vi "PlanetInfo.vi"(8 "error in (no error)":errorcluster) -> (0 "error out":errorcluster, 1 "stop?":bool, 3 "PlanetInfo":T1)   [LabVIEW 2021]
uses:
  <vilib>/Utility/miscctls.llb/LVRectTypeDef.ctl
  <vilib>/Utility/miscctls.llb/LVPoint32TypeDef.ctl
  Typedefs/PlanetInfo.ctl
  <vilib>/Utility/miscctls.llb/LVBoundsTypeDef.ctl
panel:
  out "Coords":T2
  out "Window Bounds":T3
  out "Is Window Dragged?":bool
  in  "Tab":enum32{"Page 1"}(tab)
  in  "Ring gear of teeth":dbl=72.0
  in  "Satelite gear of teeth":dbl=24.0
  in  "Sun gear of teeth":dbl=24.0
  in  "Number of satelites":dbl=3.0
  in  "Save":bool
  out "WindowHandler":bool=TRUE
  out "Komunikat":string caption="Wpisz kod"
  in  "Stop":bool
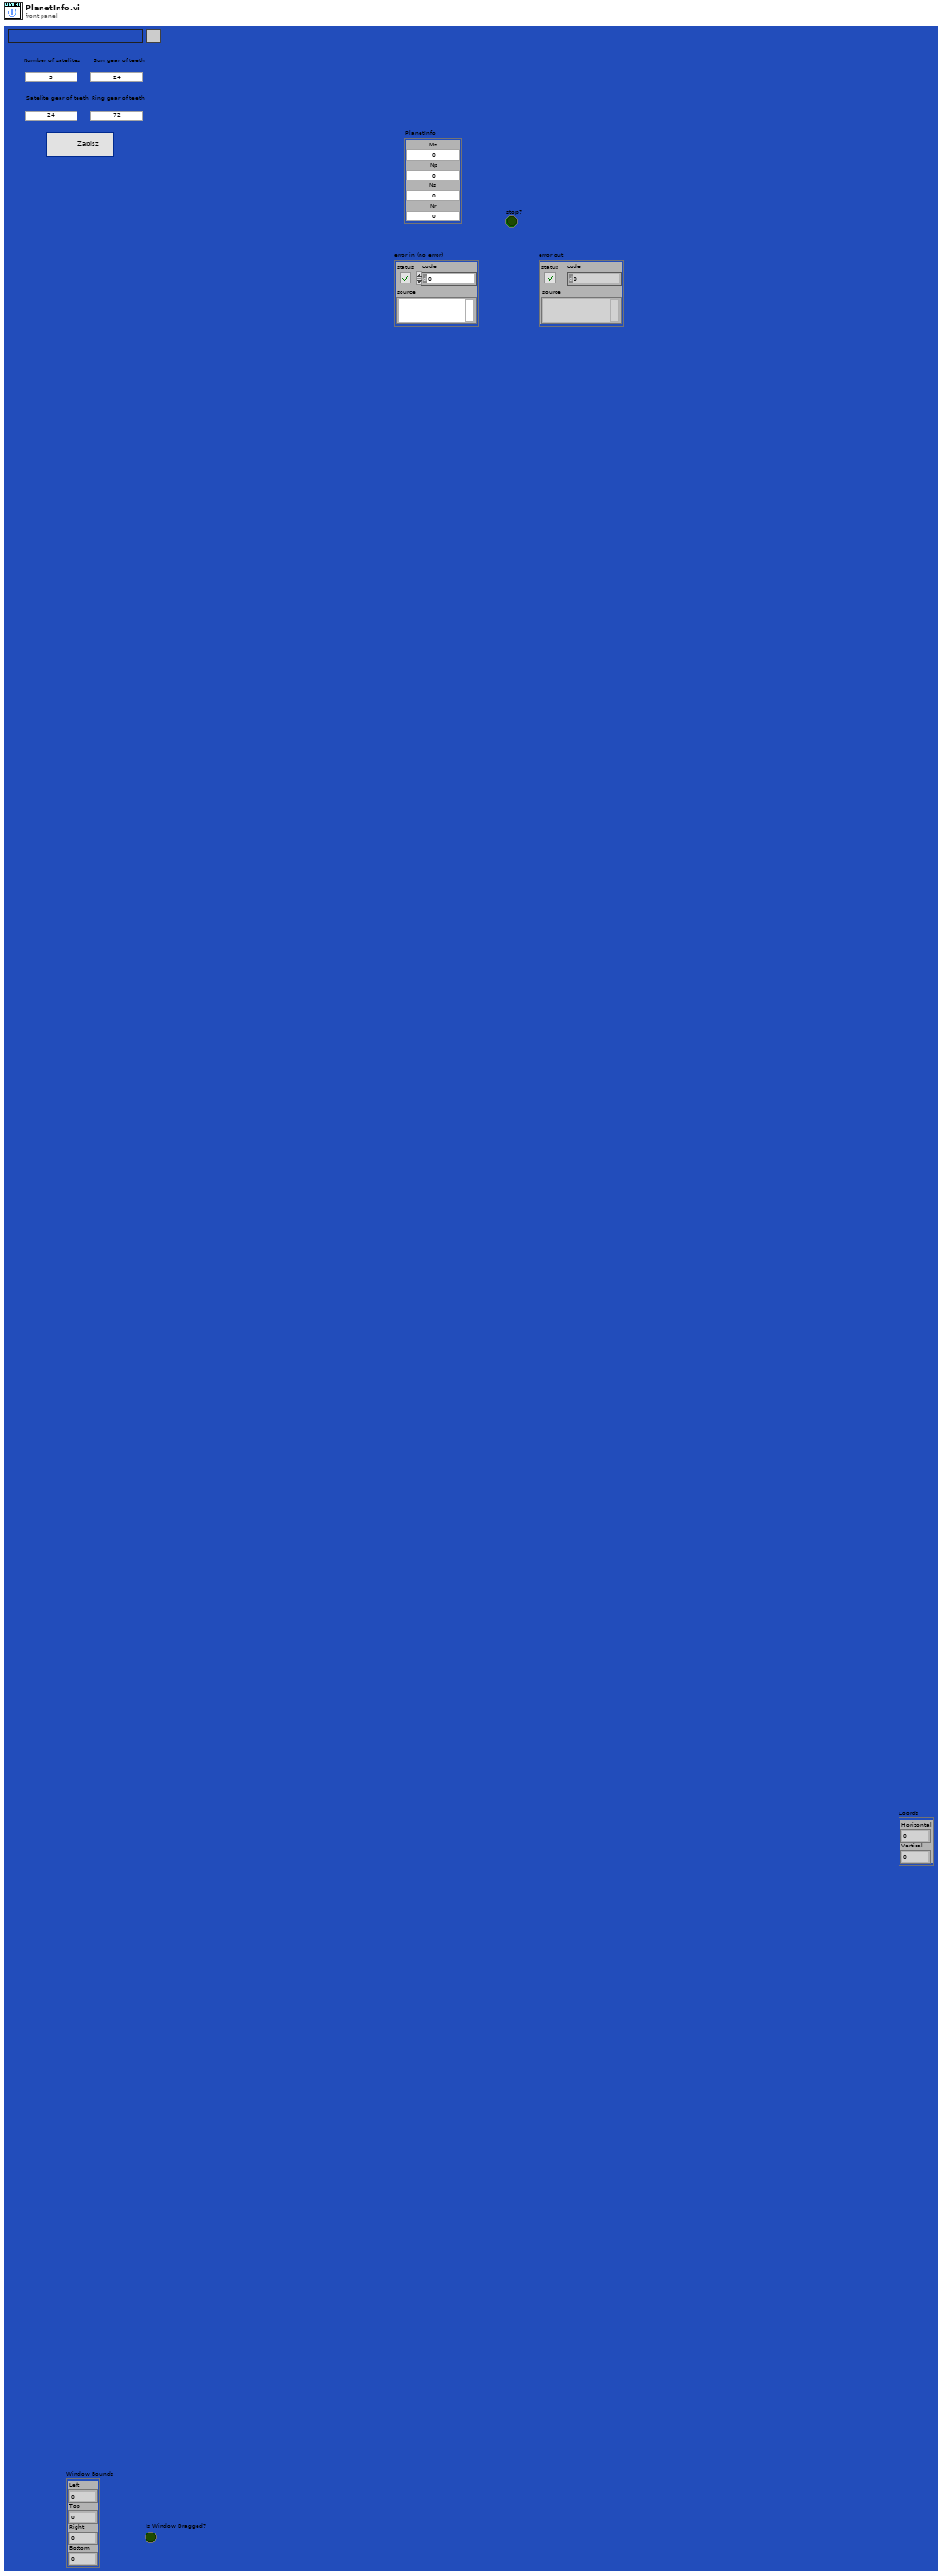
[diagram p1: front panel]
types:
  T1 = typedef "PlanetInfo.ctl" = cluster{"Ms":dbl, "Np":dbl, "Ns":dbl, "Nr":dbl}
  T2 = typedef "LVPoint32TypeDef.ctl" = cluster{"Horizontal":i32, "Vertical":i32}
  T3 = typedef "LVRectTypeDef.ctl" = cluster{"Left":i16, "Top":i16, "Right":i16, "Bottom":i16}
  T4 = typedef "LVBoundsTypeDef.ctl" = cluster{"Width":u32, "Height":u32}
  T5 = cluster{"Horizontal":i16, "Vertical":i16, "Horizontal":i16, "Vertical":i16}
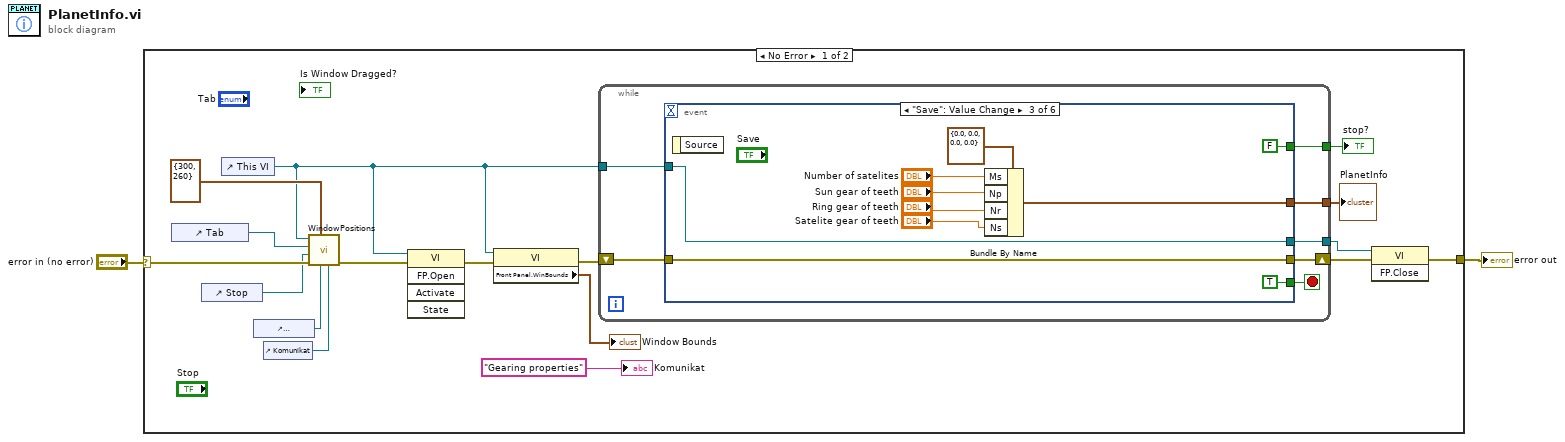
[diagram p0: block diagram]
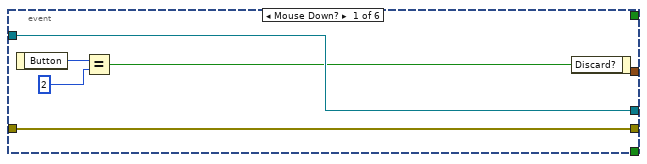
[diagram p2: hidden frame]
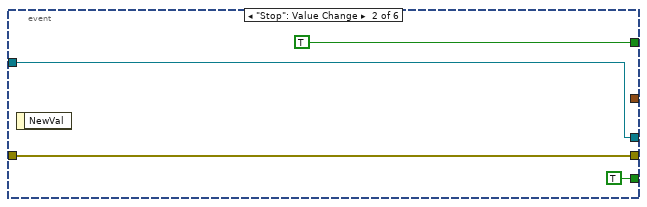
[diagram p3: hidden frame]
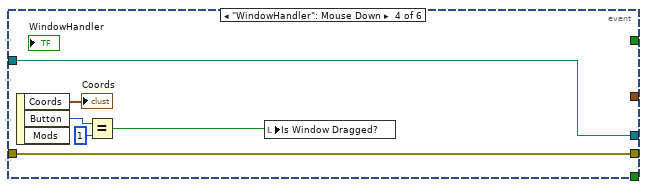
[diagram p4: hidden frame]
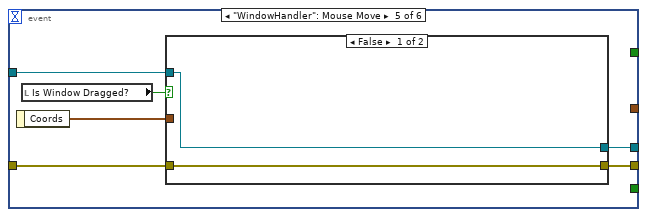
[diagram p5: hidden frame]
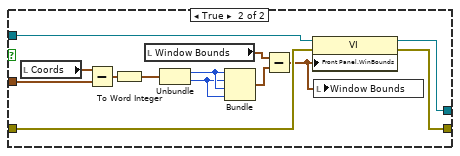
[diagram p6: hidden frame]
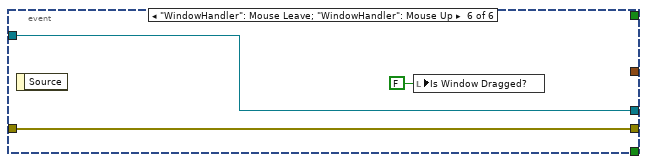
[diagram p7: hidden frame]
diagram:
  n1 = case shown="No Error" "error in (no error)" {
    selector: "error in (no error)" -> [w9 w76]
    tunnel: [w11 w76] -> w2
    frame No Error {
      n2 = control-ref of="Tab"() -> (w16:refnum<vi>)
      n3 = control-ref of="Stop"() -> (w8:refnum<vi>)
      n4 = control-ref of="This VI"() -> (w4:refnum<vi>)
      n5 = control-ref of="WindowHandler"() -> (w15:refnum<vi>)
      n6 = control-ref of="Komunikat"() -> (w14:refnum<vi>)
      n7 = call "WindowPositions.vi"("Komunikat"=w14, "WindowHandler"=w15, "Dim"=T4 {"Width"=300, "Height"=260} ("Tab Control Pane Dimension"), "error in (no error)"=w9, "Stop"=w8, "Tab"=w16, "VI in"=w4) -> ("error out"=w6:errorcluster)  [unwired: 4 in]
      n8 = invoke class="VI" method="FP.Open"(reference=w4, error in=w6) -> (error out=w5:errorcluster)  [unwired: 3 in, 4 out]
      n9 = property class="VI"(reference=w4, error in=w5) -> (error out=w19:errorcluster, "Front Panel.WinBounds"=→"Window Bounds":T3)  [unwired: 1 out]
      n10 = while {
        shift-right: [w24] -> w12
        shift-left: w19 -> [w26]
        tunnel: w4 -> [w23]
        tunnel: [w22] -> w10
        tunnel: [w21] -> w7
        tunnel: [w20] -> w3
        stop <- w25 stop-if-true
        n11 = event shown="[2] \"Save\": Value Change" {
          selector: _ -> [_ _ _ _ _ _]
          dyn-events: _ -> [_ _ _ _ _ _]
          timeout: _ -> [_ _ _ _ _ _]
          tunnel: w26 -> [w30 w34 w45 w47 w55 w74]
          tunnel: [w30 w34 w45 w47 w54 w74] -> w24
          tunnel: [_ TRUE TRUE _ _ _] -> w25
          tunnel: w23 -> [w29 w33 w43 w46 w53 w73]
          tunnel: [w29 w33 w43 w46 w52 w73] -> w22
          tunnel: [_ _ w37 _ _ _] -> w21
          tunnel: [_ TRUE ("stop? (T)") FALSE ("stop? (T)") _ _ _] -> w20
          event Mouse Down? {
            n12 = event-data() -> ("Button"=w28:u16)  [unwired: 1 in]
            n13 = Equal?(x=w28, y=u16 2) -> (x = y?=w27:bool)
            n14 = event-data("Discard?"=w27) -> ()  [unwired: 1 in, 1 out]
          }
          event "Stop": Value Change {
            n15 = event-data() -> ()  [unwired: 1 in, 1 out]
          }
          event "Save": Value Change {
            n16 = event-data() -> ()  [unwired: 1 in, 1 out]
            n17 = Bundle By Name(cluster=T1 {"Ms"=0.0, "Np"=0.0, "Ns"=0.0, "Nr"=0.0}, "Ms"="Number of satelites", "Np"="Sun gear of teeth", "Nr"="Ring gear of teeth", "Ns"="Satelite gear of teeth") -> (w37:T1)
          }
          event "WindowHandler": Mouse Down {
            n18 = event-data() -> ("Coords"=→"Coords":T2, "Button"=w50:u16)  [unwired: 1 in, 1 out]
            n19 = Equal?(x=w50, y=u16 1) -> (x = y?=w48:bool)
            n20 = local write "Is Window Dragged?"(w48) -> ()
          }
          event "WindowHandler": Mouse Move {
            n21 = event-data() -> ("Coords"=w56:T2)  [unwired: 1 in]
            n22 = local read "Is Window Dragged?"() -> (w57:bool)
            n23 = case shown="False" w57 {
              tunnel: w56 -> [_ w67]
              tunnel: w55 -> [w59 w64]
              tunnel: [w59 w63] -> w54
              tunnel: w53 -> [w58 w61]
              tunnel: [w58 w60] -> w52
              frame False {
              }
              frame True {
                n24 = local read "Coords"() -> (w68:T2)
                n25 = Subtract(x=w68, y=w67) -> (x-y=w72:T2)
                n26 = To Word Integer(number=w72) -> (16bit integer=w71:cluster{"Horizontal":i16, "Vertical":i16})
                n27 = local read "Window Bounds"() -> (w66:T3)
                n28 = Unbundle(w71) -> ("Horizontal"=w70:i16, "Vertical"=w69:i16)
                n29 = Bundle("Horizontal"=w70, "Vertical"=w69, "Horizontal"=w70, "Vertical"=w69) -> (w65:T5)  [unwired: 1 in]
                n30 = Subtract(x=w66, y=w65) -> (x-y=w62:T3)
                n31 = property class="VI"(reference=w61, error in=w64, "Front Panel.WinBounds"=w62) -> (reference out=w60:refnum<vi>, error out=w63:errorcluster)
                n32 = local write "Window Bounds"(w62) -> ()
              }
            }
          }
          event "WindowHandler": Mouse Leave; "WindowHandler": Mouse Up {
            n33 = event-data() -> ()  [unwired: 1 in, 1 out]
            n34 = local write "Is Window Dragged?"(FALSE ("Is Window Dragged?")) -> ()
          }
        }
      }
      "PlanetInfo" <- w7
      "stop?" <- w3
      n35 = invoke class="VI" method="FP.Close"(reference=w10, error in=w12) -> (error out=w11:errorcluster)  [unwired: 1 in, 2 out]
      "Komunikat" <- "Gearing properties" ("Komunikat")
    }
    frame Error {
    }
  }
  "error out" <- w2
